vi "Capture UI State [UIM].vi"(6 "Variant in":variant, 7 "Shift Pressed?":bool, 8 "error in (no error)":errorcluster, 10 "QD Combo Box Ref":refnum<vi>, 11 "QD Launch VI Ref":refnum<vi>) -> (0 "error out":errorcluster, 4 "Variant out":variant)   [LabVIEW 2015]
doc: "Captures the current UI state, using the User Interface Manager API, into an XML file with the same name as the current VI and next to it. If you use the <Shift> while you use this QuickDrop shortcut the text typed in the QuickDrop ComboBox will be used as the captured state name.\n\nDefault Shortcut - [U]"
panel:
  in  "Undo Name":string="Insert"
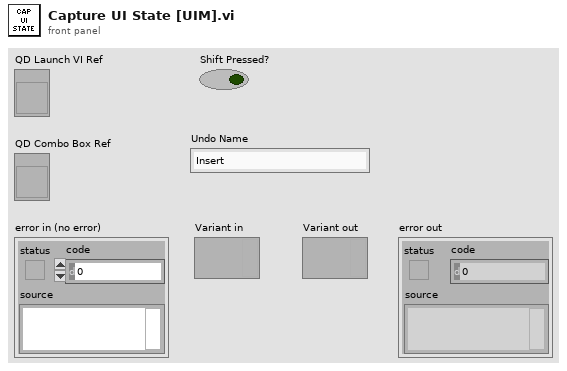
[diagram p1: front panel]
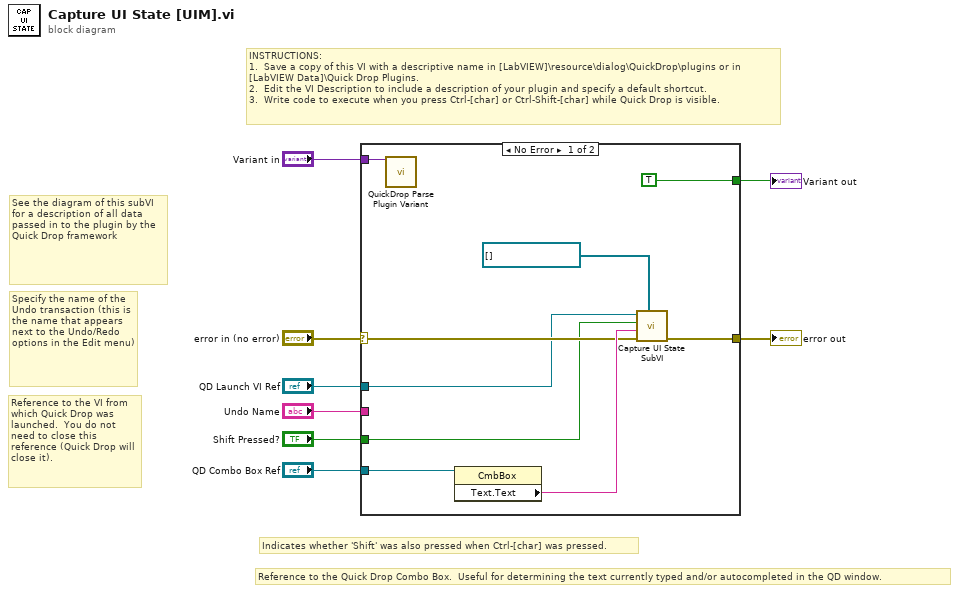
[diagram p0: block diagram]
diagram:
  # "See the diagram of this subVI for a description of all data passed in to the plugin by the Quick Drop framework"
  # "Reference to the Quick Drop Combo Box.  Useful for determining the text currently typed and/or autocompleted in the QD window."
  # "Indicates whether 'Shift' was also pressed when Ctrl-[char] was pressed."
  # "Specify the name of the Undo transaction (this is the name that appears next to the Undo/Redo options in the Edit menu)"
  # "Reference to the VI from which Quick Drop was launched.  You do not need to close this reference (Quick Drop will close it)."
  # "INSTRUCTIONS:\n1.  Save a copy of this VI with a descriptive name in [LabVIEW]\\resource\\dialog\\QuickDrop\\plugins or in [LabVIEW Data]\\Quick Drop Plugins.\n2.  Edit the VI Description to include a description of your plugin and specify a default shortcut. \n3.  Write code to execute when you press Ctrl-[char] or Ctrl-Shift-[char] while Quick Drop is visible."
  n1 = case shown="No Error" "error in (no error)" {
    selector: "error in (no error)" -> [w13 w18]
    tunnel: [w12 w18] -> w2
    tunnel: "QD Launch VI Ref" -> [w11 _]
    tunnel: "Shift Pressed?" -> [w9 _]
    tunnel: "QD Combo Box Ref" -> [w15 _]
    tunnel: "Variant in" -> [w17 _]
    tunnel: "Undo Name" -> [_ _]
    tunnel: [TRUE _] -> w1
    frame No Error {
      n2 = call <vilib>:"QuickDrop Parse Plugin Variant.vi"("QDKS Variant in"=w17) -> ()  [unwired: 12 in, 3 out]
      n3 = property class="CmbBox"(reference=w15) -> ("Text.Text"=w14:string)  [unwired: 1 in, 2 out]
      n4 = call "Capture UI State SubVI.vi"("Ctls Refs (All Ctls)"=refnum<vi>[] [], "error in (no error)"=w13, "ComboBox Text"=w14, "Shift Pressed"=w9, "VI Ref In"=w11) -> ("error out"=w12:errorcluster)  [unwired: 6 in]
    }
    frame Error {
    }
  }
  "error out" <- w2
  "Variant out" <- w1
